vi "After Launch Init.vi"(8 "error in (no error)":errorcluster, 11 "CS++DCPwr in":refnum<class "CS++DCPwr.lvclass">) -> (0 "error out":errorcluster, 3 "CS++DCPwr out":refnum<class "CS++DCPwr.lvclass">)   [LabVIEW 2013, in "CS++DCPwr.lvlib" / "CS++DCPwr.lvclass"]
doc: "Use <b>Pre Launch init.vi</b> method for sanity checks that are supposed to prevent the actor from launching if they fail. Use <B>this</B> method instead to initialize this actor when it has been activated. A corresponding high priority message will become dispatched before the <B>Actor Core.vi</b> is called.\n\nRefer also to the ongoing discussion at https://decibel.ni.com/content/message/57394#57394."
uses:
  CS++DCPwr.lvclass
  CSPP_Core/Classes/CS++ProcessVariables/ProcessVariable/PV.lvclass
  CSPP_Core/Classes/CS++ProcessVariables/SVConnection/SVConnection.lvclass
  CS++DCPwr.lvclass/CS++DCPwr.ctl
  CSPP_Core/Classes/CS++ProcessVariables/ProcessVariable/PV.lvclass/PV.ctl
  CSPP_Core/Classes/CS++ProcessVariables/PVConnection/PVConnection.lvclass/PVConnection.ctl
  CSPP_Core/Actors/CS++DeviceActor/CS++DeviceActor.lvclass
  CSPP_Core/Actors/CS++DeviceActor/CS++DeviceActor.lvclass/CS++DeviceActor.ctl
  CS++DCPwr Messages/Measure [MSR] Msg/Measure [MSR] Msg.lvclass
  <vilib>/ActorFramework/Actor/Actor.lvclass/Actor.ctl
  <vilib>/ActorFramework/Message Enqueuer/Message Enqueuer.lvclass/Message Enqueuer.ctl
  CS++DCPwr Messages/Measure [MSR] Msg/Measure [MSR] Msg.lvclass/Measure [MSR] Msg.ctl
  CS++DCPwr Messages/Measure [MSR] Msg/Write channel name.vi
  CS++DCPwr Messages/Measure [MSR] Msg/Write measurement type.vi
  CSPP_Core/Classes/CS++ProcessVariables/ProcessVariable/Write PV URL.vi
  CSPP_Core/Classes/CS++ProcessVariables/ProcessVariable/Write Data.vi
  CSPP_Core/Classes/CS++ProcessVariables/ProcessVariable/Write Error.vi
  CSPP_Core/Classes/CS++ProcessVariables/ProcessVariable/Write Quality.vi
  CSPP_Core/Classes/CS++ProcessVariables/ProcessVariable/Write status.vi
  CSPP_Core/Classes/CS++ProcessVariables/ProcessVariable/Write Timestamp.vi
  CSPP_Core/Classes/CS++ProcessVariables/PVConnection/Write PV URL.vi
  <vilib>/ActorFramework/Message Enqueuer/Init from Existing Queue.vi
  <vilib>/ActorFramework/Message Enqueuer/Message Enqueuer.lvclass
  <vilib>/ActorFramework/Actor/Actor.lvclass
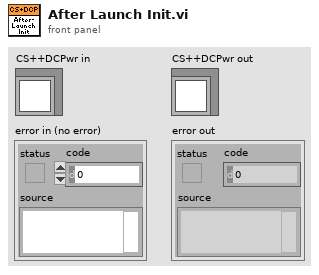
[diagram p1: front panel]
types:
  T1 = cluster{"Write Access":enum8{"Allowed", "Required", "None"}, "Read Access":enum8{"Allowed", "Required", "None"}}
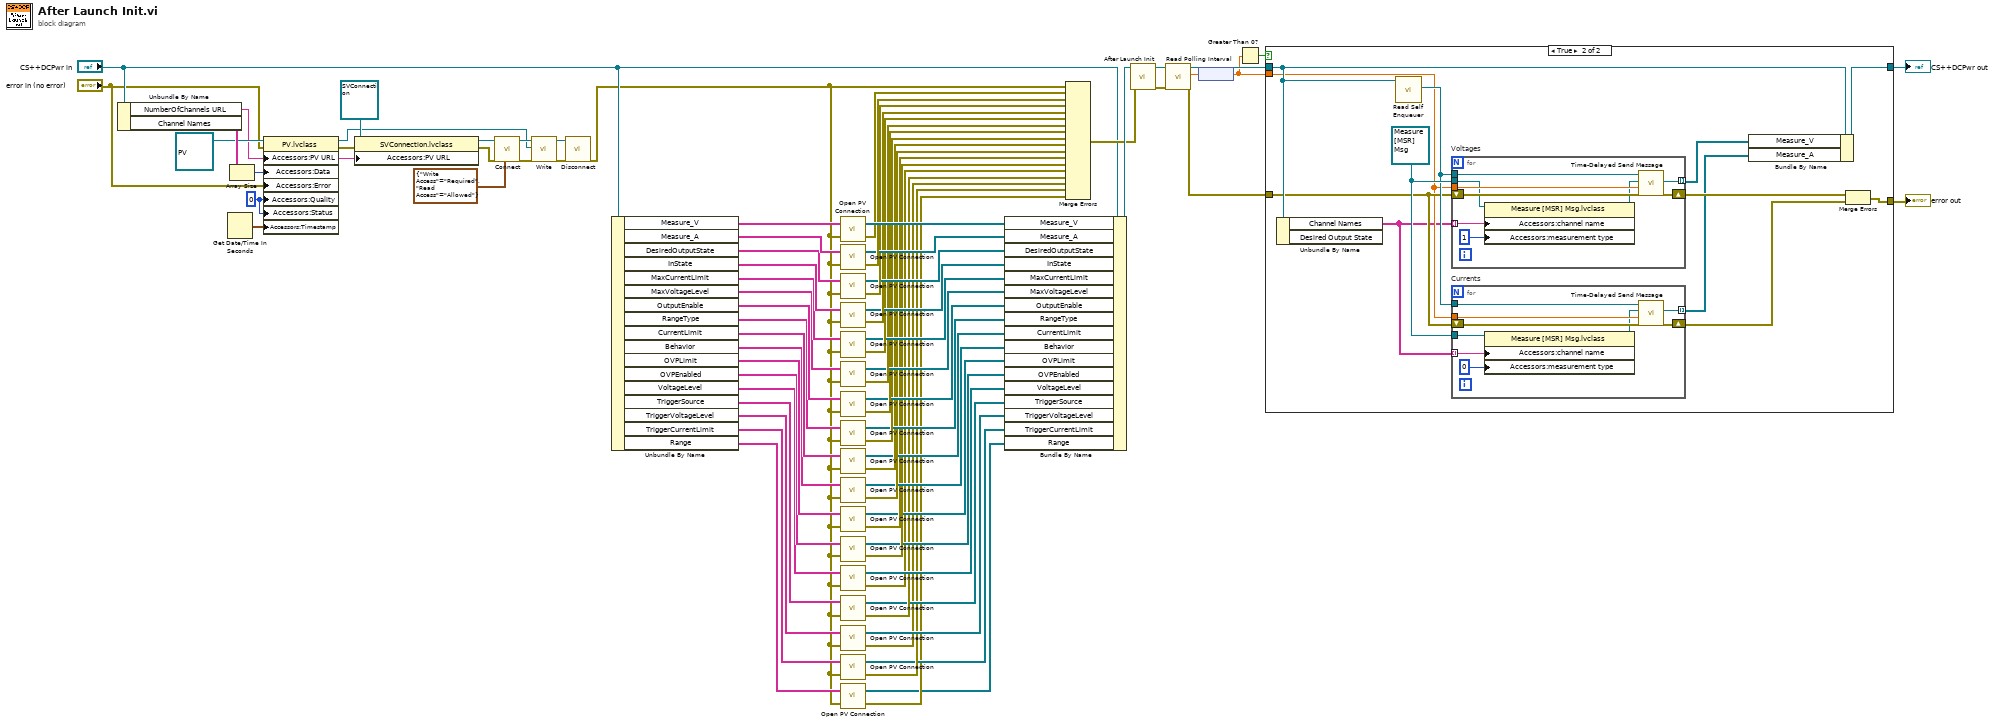
[diagram p0: block diagram]
diagram:
  w18 = 0 ("Quality")
  n1 = Unbundle By Name("CS++DCPwr in") -> ("NumberOfChannels URL"=w14:string, "Channel Names"=w22:string[])
  n2 = Get Date/Time In Seconds() -> (seconds since 1Jan1904=w17:timestamp)
  n3 = Array Size(array=w22) -> (size(s)=w20:i32)
  n4 = property class="PV.lvclass"(reference=refnum<class "PV.lvclass"> refnum ("CS++ProcessVariables.lvlib:PV.lvclass"), error in="error in (no error)", "Accessors:PV URL"=w14, "Accessors:Data"=w20, "Accessors:Error"="error in (no error)", "Accessors:Quality"=w18, "Accessors:Status"=w18, "Accessors:Timestamp"=w17) -> (reference out=w8:refnum<class "PV.lvclass">, error out=w13:errorcluster)
  n5 = property class="SVConnection.lvclass"(reference=refnum<class "SVConnection.lvclass"> refnum ("CS++ProcessVariables.lvlib:SVConnection.lvclass"), error in=w13, "Accessors:PV URL"=w14) -> (reference out=w15:refnum<class "SVConnection.lvclass">, error out=w12:errorcluster)
  n6 = call-dynamic "Connect.vi"("Access"=T1 {"Write Access"=enum."Required", "Read Access"=enum."Allowed"}, "error in (no error)"=w12, "PVConnection in"=w15) -> ("error out"=w9:errorcluster, "PVConnection out"=w10:refnum<class "SVConnection.lvclass">)  [unwired: 7 in]
  n7 = call-dynamic "Write.vi"("error in (no error)"=w9, "PV"=w8, "PVConnection in"=w10) -> ("error out"=w6:errorcluster, "PVConnection out"=w7:refnum<class "SVConnection.lvclass">)  [unwired: 7 in]
  n8 = call-dynamic "Disconnect.vi"("error in (no error)"=w6, "PVConnection in"=w7) -> ("error out"=w3:errorcluster)  [unwired: 8 in, 1 out]
  n9 = Unbundle By Name("CS++DCPwr in") -> ("Measure_V"=w70:string[], "Measure_A"=w63:string[], "DesiredOutputState"=w62:string[], "InState"=w61:string[], "MaxCurrentLimit"=w58:string[], "MaxVoltageLevel"=w53:string[], "OutputEnable"=w52:string[], "RangeType"=w49:string[], "CurrentLimit"=w46:string[], "Behavior"=w45:string[], "OVPLimit"=w40:string[], "OVPEnabled"=w39:string[], "VoltageLevel"=w34:string[], "TriggerSource"=w31:string[], "TriggerVoltageLevel"=w26:string[], "TriggerCurrentLimit"=w23:string[], "Range"=w4:string[])
  n10 = call "Open PV Connection.vi"("Error In"=w3, "URLs"=w70) -> ("Error Out"=w68:errorcluster, "PV Connections"=w69:refnum<class "SVConnection.lvclass">[])
  n11 = call "Open PV Connection.vi"("Error In"=w3, "URLs"=w63) -> ("Error Out"=w67:errorcluster, "PV Connections"=w66:refnum<class "SVConnection.lvclass">[])
  n12 = call "Open PV Connection.vi"("Error In"=w3, "URLs"=w62) -> ("Error Out"=w65:errorcluster, "PV Connections"=w64:refnum<class "SVConnection.lvclass">[])
  n13 = call "Open PV Connection.vi"("Error In"=w3, "URLs"=w61) -> ("Error Out"=w60:errorcluster, "PV Connections"=w59:refnum<class "SVConnection.lvclass">[])
  n14 = call "Open PV Connection.vi"("Error In"=w3, "URLs"=w58) -> ("Error Out"=w57:errorcluster, "PV Connections"=w56:refnum<class "SVConnection.lvclass">[])
  n15 = call "Open PV Connection.vi"("Error In"=w3, "URLs"=w53) -> ("Error Out"=w55:errorcluster, "PV Connections"=w54:refnum<class "SVConnection.lvclass">[])
  n16 = call "Open PV Connection.vi"("Error In"=w3, "URLs"=w52) -> ("Error Out"=w51:errorcluster, "PV Connections"=w50:refnum<class "SVConnection.lvclass">[])
  n17 = call "Open PV Connection.vi"("Error In"=w3, "URLs"=w49) -> ("Error Out"=w48:errorcluster, "PV Connections"=w47:refnum<class "SVConnection.lvclass">[])
  n18 = call "Open PV Connection.vi"("Error In"=w3, "URLs"=w46) -> ("Error Out"=w44:errorcluster, "PV Connections"=w42:refnum<class "SVConnection.lvclass">[])
  n19 = call "Open PV Connection.vi"("Error In"=w3, "URLs"=w45) -> ("Error Out"=w43:errorcluster, "PV Connections"=w41:refnum<class "SVConnection.lvclass">[])
  n20 = call "Open PV Connection.vi"("Error In"=w3, "URLs"=w40) -> ("Error Out"=w38:errorcluster, "PV Connections"=w36:refnum<class "SVConnection.lvclass">[])
  n21 = call "Open PV Connection.vi"("Error In"=w3, "URLs"=w39) -> ("Error Out"=w37:errorcluster, "PV Connections"=w35:refnum<class "SVConnection.lvclass">[])
  n22 = call "Open PV Connection.vi"("Error In"=w3, "URLs"=w34) -> ("Error Out"=w32:errorcluster, "PV Connections"=w33:refnum<class "SVConnection.lvclass">[])
  n23 = call "Open PV Connection.vi"("Error In"=w3, "URLs"=w31) -> ("Error Out"=w30:errorcluster, "PV Connections"=w29:refnum<class "SVConnection.lvclass">[])
  n24 = call "Open PV Connection.vi"("Error In"=w3, "URLs"=w26) -> ("Error Out"=w27:errorcluster, "PV Connections"=w28:refnum<class "SVConnection.lvclass">[])
  n25 = call "Open PV Connection.vi"("Error In"=w3, "URLs"=w23) -> ("Error Out"=w25:errorcluster, "PV Connections"=w24:refnum<class "SVConnection.lvclass">[])
  n26 = call "Open PV Connection.vi"("Error In"=w3, "URLs"=w4) -> ("Error Out"=w2:errorcluster, "PV Connections"=w1:refnum<class "SVConnection.lvclass">[])
  n27 = Bundle By Name(cluster="CS++DCPwr in", "Measure_V"=w69, "Measure_A"=w66, "DesiredOutputState"=w64, "InState"=w59, "MaxCurrentLimit"=w56, "MaxVoltageLevel"=w54, "OutputEnable"=w50, "RangeType"=w47, "CurrentLimit"=w42, "Behavior"=w41, "OVPLimit"=w36, "OVPEnabled"=w35, "VoltageLevel"=w33, "TriggerSource"=w29, "TriggerVoltageLevel"=w28, "TriggerCurrentLimit"=w24, "Range"=w1) -> (w81:refnum<class "CS++DCPwr.lvclass">)
  n28 = Merge Errors(w3, w68, w67, w65, w60, w57, w55, w51, w48, w44, w43, w38, w37, w32, w30, w27, w25, w2) -> (w80:errorcluster)
  n29 = call-parent "After Launch Init.vi"("error in (no error)"=w80, "CS++DeviceActor in"=w81) -> ("error out"=w77:errorcluster, "CS++DeviceActor out"=w79:refnum<class "CS++DCPwr.lvclass">)  [unwired: 8 in]
  n30 = call "Read Polling Interval.vi"("error in (no error)"=w77, "CS++DeviceActor in"=w79) -> ("error out"=w76:errorcluster, "Polling Interval"=w75:dbl[unit], "CS++DeviceActor out"=w78:refnum<class "CS++DCPwr.lvclass">)  [unwired: 7 in]
  n31 = node(w75) -> (w74:dbl)
  n32 = Greater Than 0?(x=w74) -> (x > 0?=w73:bool)
  n33 = case shown="True" w73 {
    tunnel: [w83 w95] -> w72
    tunnel: [w82 w93] -> w71
    tunnel: w78 -> [w83 w94]
    tunnel: w76 -> [w82 w86]
    tunnel: w74 -> [_ w85]
    frame False {
    }
    frame True {
      w88 = refnum<class "Measure [MSR] Msg.lvclass"> refnum ("CS++DCPwr.lvlib:Measure [MSR] Msg.lvclass")
      n34 = Unbundle By Name(w94) -> ("Channel Names"=w84:string[])  [unwired: 1 out]
      n35 = call <vilib>:"Read Self Enqueuer.vi"("Actor"=w94) -> ("Self Enqueuer"=w87:refnum<class "Message Enqueuer.lvclass">)  [unwired: 10 in]
      n36 = for "Voltages" {
        tunnel: w87 -> [w112]
        tunnel: w85 -> [w110]
        tunnel: [w109] -> w91 mode=indexing
        tunnel: w88 -> [w105]
        shift-right: [w113] -> w92
        shift-left: w86 -> [w111]
        tunnel: w84 -> [w108] mode=indexing
        n37 = property class="Measure [MSR] Msg.lvclass"(reference=w105, "Accessors:channel name"=w108, "Accessors:measurement type"=1 ("measurement type (voltage)")) -> (reference out=w106:refnum<class "Measure [MSR] Msg.lvclass">)  [unwired: 1 in, 1 out]
        n38 = call <vilib>:"Time-Delayed Send Message.vi"("error in (no error)"=w111, "Milliseconds To Wait"=w110, "Message"=w106, "Message Enqueuer"=w112) -> ("error out"=w113:errorcluster, "Delivery Notifier"=w109:refnum<notifier>)  [unwired: 6 in]
      }
      n39 = for "Currents" {
        tunnel: w87 -> [w103]
        tunnel: w85 -> [w101]
        tunnel: [w100] -> w90 mode=indexing
        shift-right: [w104] -> w89
        shift-left: w86 -> [w102]
        tunnel: w84 -> [w99] mode=indexing
        tunnel: w88 -> [w96]
        n40 = property class="Measure [MSR] Msg.lvclass"(reference=w96, "Accessors:channel name"=w99, "Accessors:measurement type"=0 ("measurement type (voltage)")) -> (reference out=w97:refnum<class "Measure [MSR] Msg.lvclass">)  [unwired: 1 in, 1 out]
        n41 = call <vilib>:"Time-Delayed Send Message.vi"("error in (no error)"=w102, "Milliseconds To Wait"=w101, "Message"=w97, "Message Enqueuer"=w103) -> ("error out"=w104:errorcluster, "Delivery Notifier"=w100:refnum<notifier>)  [unwired: 6 in]
      }
      n42 = Bundle By Name(cluster=w94, "Measure_V"=w91, "Measure_A"=w90) -> (w95:refnum<class "CS++DCPwr.lvclass">)
      n43 = Merge Errors(w92, w89) -> (w93:errorcluster)
    }
  }
  "error out" <- w71
  "CS++DCPwr out" <- w72
